vi "_memcpy.vi"(0 "MDPtr DVR":refnum<data-value>, 1 "Copy Count":i32, 5 "error in (no error)":errorcluster, 7 "Memory":string, 9 "String Attribute":string, 12 "Data Type":T1) -> (4 "MDPtr DVR(dup)":refnum<data-value>, 6 "error out":errorcluster)   [LabVIEW 2017, in "MDPtr.lvlib"]
uses:
  MDPtr.lvlib
  MDPtr TypeDef/MDPtr DataFrame-Memory.ctl
  MDPtr TypeDef/MDPtr DataFrame-Common.ctl
  <vilib>/Utility/Data Type/Type Definitions/Data Type.ctl
  Error Handler/_Build Error Cluster.vi
  <vilib>/Utility/Data Type/NI_Data Type.lvlib
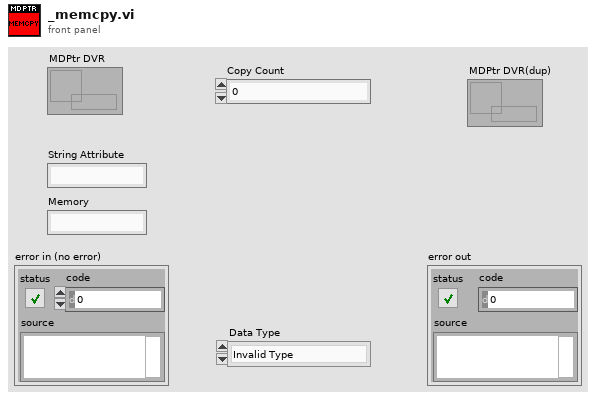
[diagram p1: front panel]
types:
  T1 = typedef "NI_Data Type.lvlib/Data Type.ctl" = enum8{"Invalid Type", "Void", "I8", "I16", "I32", "I64", "U8", "U16", "U32", "U64", "Single Float", "Double Float", "Extended Float", "Single Complex", "Double Complex", "Extended Complex", "Enum U8", "Enum U16", "Enum U32", "Enum U64", "Single Float With Unit", "Double Float With Unit", "Extended Float With Unit", "Single Complex with Unit", "Double Complex with Unit", "Extended Complex with Unit", "Boolean", "String", "Path", "Picture", "Tag", "Array", "Cluster", "Variant", "LV Variant", "Waveform", "Timestamp", "Digital Waveform", "Digital Data", "ExpressData", "Refnum", "External Data", "VI", "Poly VI", "LabVIEW Class Instance", "Fixed Point"}
  T2 = typedef "MDPtr.lvlib/MDPtr DataFrame-Memory.ctl" = cluster{"Common":T3, "DVR":refnum<data-value>}
  T3 = typedef "MDPtr.lvlib/MDPtr DataFrame-Common.ctl" = cluster{"Data Type":T1, "Copy Count":i32, "String Attribute":string, "Cache Length":i32, "Data Length":i32}
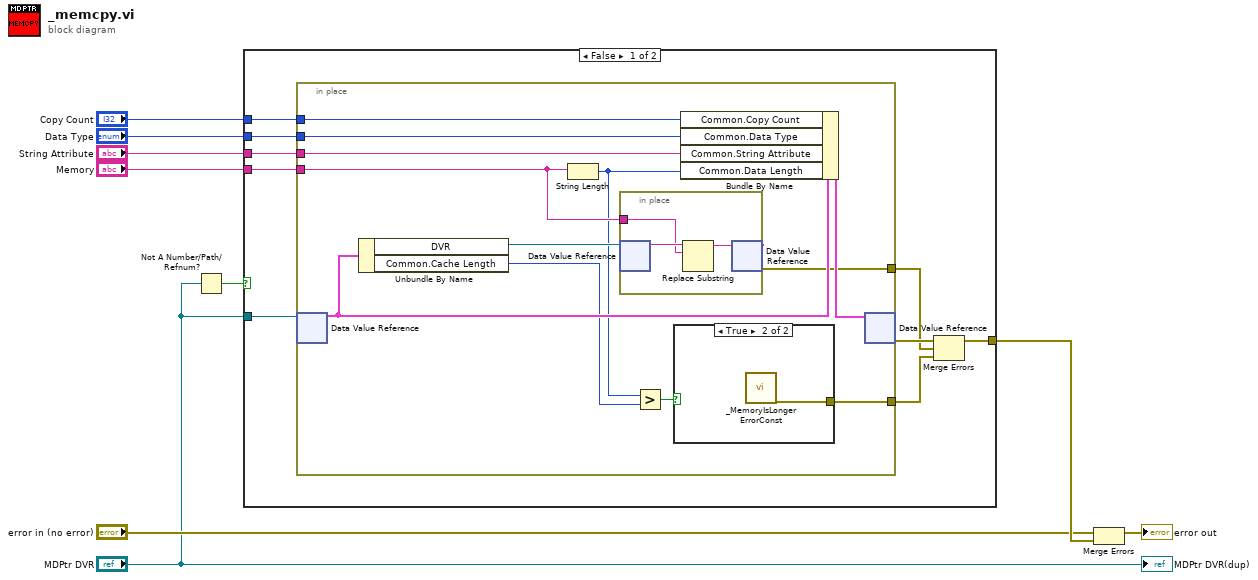
[diagram p0: block diagram]
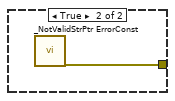
[diagram p3: hidden frame]
diagram:
  n1 = Not A Number/Path/Refnum?(number/path/refnum="MDPtr DVR") -> (NaN/Path/Refnum?=w5:bool)
  n2 = case shown="False" w5 {
    tunnel: [w12 w35] -> w9
    tunnel: "MDPtr DVR" -> [w17 _]
    tunnel: "Copy Count" -> [w16 _]
    tunnel: "Data Type" -> [w15 _]
    tunnel: "String Attribute" -> [w14 _]
    tunnel: "Memory" -> [w13 _]
    frame False {
      n3 = in-place {
        in-place-border: w16 -> [w29]
        in-place-border: w15 -> [w28]
        in-place-border: w14 -> [w27]
        in-place-border: w13 -> [w23]
        in-place-border: [w24] -> w11
        in-place-border: [w19] -> w10
        n4 = in-place-dvr #1(w17) -> (w26:T2)  [unwired: 1 out]
        n5 = Unbundle By Name(w26) -> ("DVR"=w25:refnum<data-value>, "Common.Cache Length"=w21:i32)
        n6 = String Length(string=w23) -> (length=w22:i32)
        n7 = in-place {
          in-place-border: w23 -> [w32]
          n8 = in-place-dvr #2(w25) -> (w34:string)  [unwired: 1 out]
          n9 = Replace Substring(4:w32, 5:w34) -> (1:w33:string)  [unwired: 2 in, 1 out]
          n10 = in-place-dvr #2(w33) -> (w24:errorcluster)  [unwired: 1 out]
        }
        n11 = Greater?(x=w22, y=w21) -> (0:w20:bool)
        n12 = case shown="True" w20 {
          tunnel: [_ w31] -> w19
          frame False {
          }
          frame True {
            n13 = call "_MemoryIsLonger ErrorConst.vi"() -> ("error out"=w31:errorcluster)  [unwired: 19 in]
          }
        }
        n14 = Bundle By Name(cluster=w26, "Common.Copy Count"=w29, "Common.Data Type"=w28, "Common.String Attribute"=w27, "Common.Data Length"=w22) -> (w30:T2)
        n15 = in-place-dvr #1(w30) -> (w18:errorcluster)  [unwired: 1 out]
      }
      n16 = Merge Errors(w18, w11, w10) -> (w12:errorcluster)
    }
    frame True {
      n17 = call "_NotValidStrPtr ErrorConst.vi"() -> ("error out"=w35:errorcluster)  [unwired: 19 in]
    }
  }
  n18 = Merge Errors("error in (no error)", w9) -> (→"error out":errorcluster)
  "MDPtr DVR(dup)" <- "MDPtr DVR"
